vi "mh.vi"(5 "Connectivity":bool, 7 "Image Src":T1, 9 "Fill Value":u8, 11 "error in (no error)":errorcluster, 12 "Tolerance":sgl, 13 "Hot spot (x,y)":i32[](array[numeric])) -> (4 "Refnum out":T1, 6 "ROI Descriptor":T3 {"Contours"."Type" items=["No Selection", "Point", "Line", "Rectangle", "Oval", "Polygon", "Freehand Region", "Annulus", "Unused2", "Unused3", "Broken Line", "Freehand Line", "Rotated Rectangle"]}, 10 "Statistics":T2, 14 "Histograms":u32[][](array[numeric]), 15 "error out":errorcluster)   [LabVIEW 2020]
uses:
  <vilib>/vision/Image Controls.llb/IMAQ Image.ctl
  <vilib>/vision/NI_Vision_Development_Module.lvlib
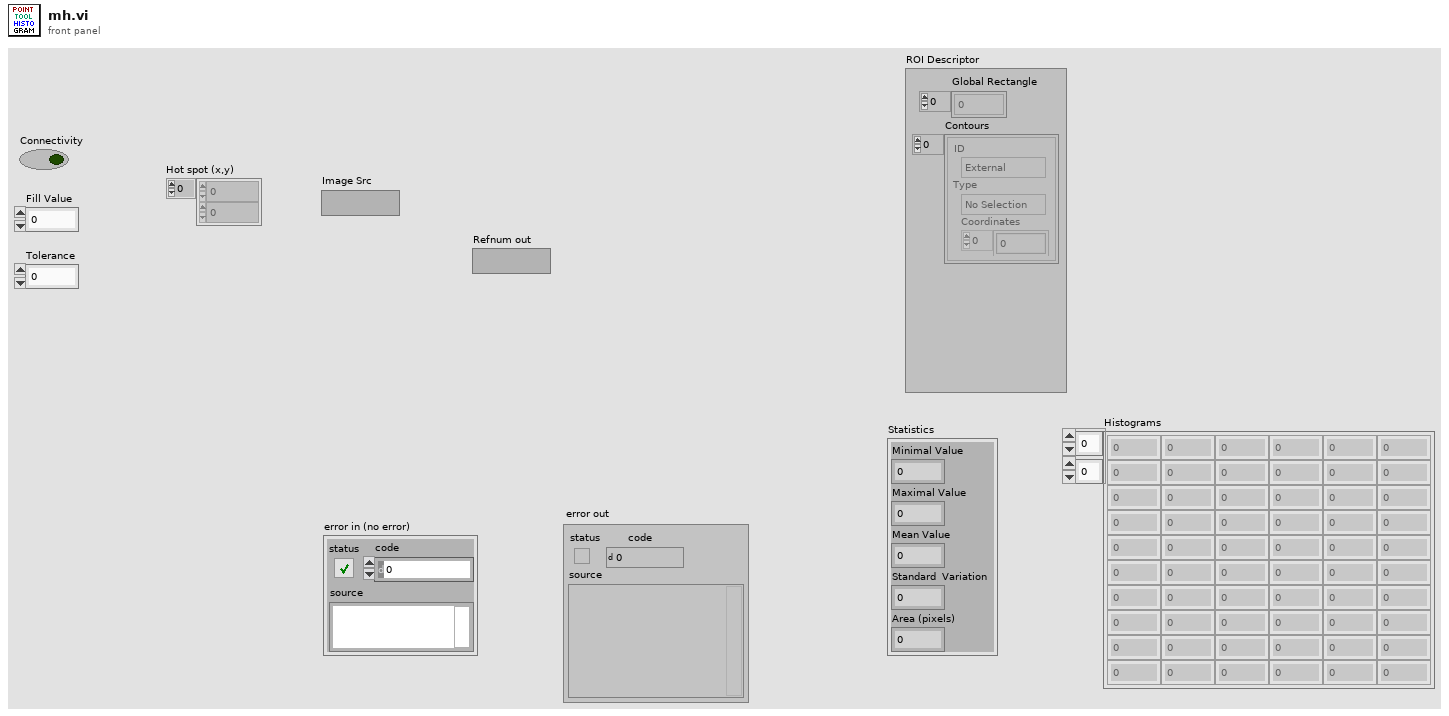
[diagram p1: front panel]
types:
  T1 = typedef "IMAQ Image.ctl" = refnum<image>
  T2 = cluster{"Minimal Value":sgl, "Maximal Value":sgl, "Mean Value":sgl, "Standard  Variation":sgl, "Area (pixels)":i32}
  T3 = typedef "ROI Descriptor" = cluster{"Global Rectangle":i32[], "Contours":cluster{"ID":enum32{"External", "Internal"}, "Type":u32, "Coordinates":i32[]}[]}
  T4 = typedef "Image Type" = u32
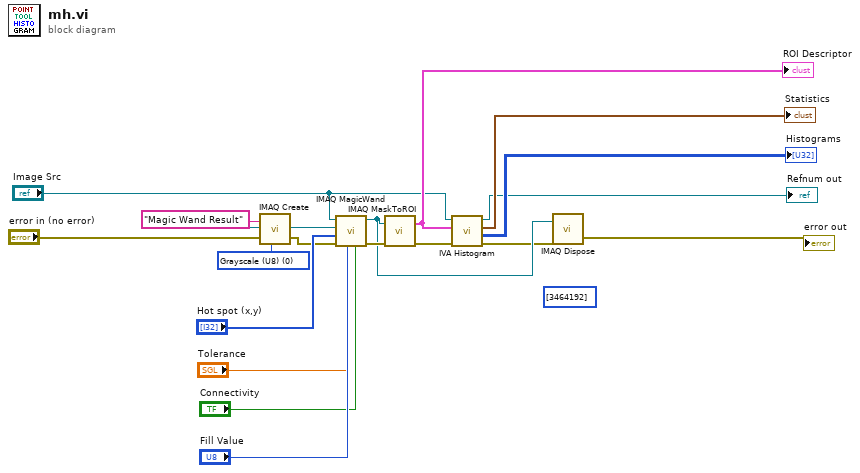
[diagram p0: block diagram]
diagram:
  w9 = T4 0 items=["Grayscale (U8)", "Grayscale (I16)", "Grayscale (SGL)", "Complex (CSG)", "RGB (U32)", "HSL (U32)", "RGB (U64)", "Grayscale (U16)"] ("Image Type")
  (unwired) u32[] [3464192] ("Colors (Green)")
  n1 = call "IMAQ Create"("Image Name"="Magic Wand Result", "Image Type"=w9, "error in (no error)"="error in (no error)") -> ("New Image"=w5:T1, "error out"=w8:errorcluster)  [unwired: 2 in]
  n2 = call "IMAQ MagicWand"("Connectivity 4/8 (8)"="Connectivity", "Tolerance"="Tolerance", "Fill Value"="Fill Value", "error in (no error)"=w8, "Hot spot (x,y)"="Hot spot (x,y)", "Image Dst"=w5, "Image Src"="Image Src") -> ("error out"=w15:errorcluster, "Image Dst Out"=w3:T1)  [unwired: 3 in]
  n3 = call "IMAQ MaskToROI"("Image"=w3, "error in (no error)"=w15) -> ("ROI Descriptor"=w18:T3, "error out"=w19:errorcluster)  [unwired: 5 in, 1 out]
  "ROI Descriptor" <- w18
  n4 = call <vilib>:"IVA Histogram.vi"("error in (no error)"=w19, "ROI Descriptor"=w18, "Image In"="Image Src") -> ("error out"=w1:errorcluster, "Histograms"=→"Histograms":u32[][], "Statistics"=→"Statistics":T2, "Image Out"=→"Refnum out":T1)  [unwired: 1 in, 4 out]
  n5 = call "IMAQ Dispose"("Image"=w3, "error in (no error)"=w1) -> ("error out"=→"error out":errorcluster)  [unwired: 4 in]
